vi "WS1050 Dec to Hex.vi"(8 "error in (no error)":errorcluster) -> (0 "error out":errorcluster, 3 "Hex":string[](array[string]))   [LabVIEW 2012]
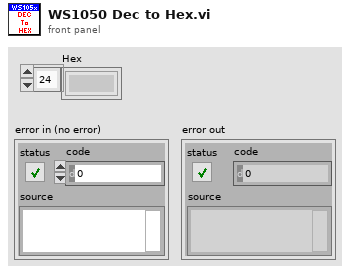
[diagram p1: front panel]
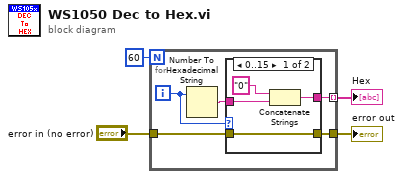
[diagram p0: block diagram]
diagram:
  n1 = for {
    N: 60 -> [_]
    tunnel: [w6] -> w3 mode=indexing
    tunnel: "error in (no error)" -> [w9]
    tunnel: [w8] -> w1
    i -> [w7]
    n2 = Number To Hexadecimal String(2:w7) -> (0:w5:string)  [unwired: 1 in]
    n3 = case shown="0..15" w7 {
      tunnel: w9 -> [w10 w15]
      tunnel: [w10 w15] -> w8
      tunnel: [w13 w14] -> w6
      tunnel: w5 -> [w12 w14]
      frame 0..15 {
        n4 = Concatenate Strings("0" ("string"), w12) -> (w13:string)
      }
      frame 16, Default {
      }
    }
  }
  "Hex" <- w3
  "error out" <- w1
